vi "Turn Saunders Chamber Off2023.vi"(2 "error in":errorcluster, 3 "Mode":u8 max=2 step=1, 4 "GPIB#":u8=1 max=4 step=1, 5 "GPIB Address":u8=2 max=30 step=1) -> (0 "error out":errorcluster)   [LabVIEW 2023]
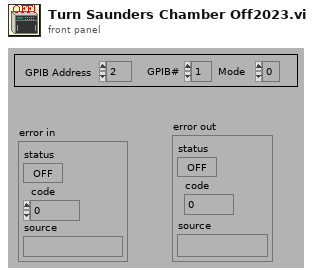
[diagram p1: front panel]
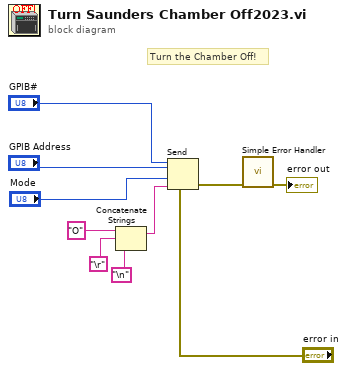
[diagram p0: block diagram]
diagram:
  # "Turn the Chamber Off!"
  n1 = Concatenate Strings("O" ("data string"), "\r", "\n") -> (w3:string)
  n2 = Send(0:"GPIB#", 2:"GPIB Address", 3:"Mode", 4:"error in", 5:w3) -> (8:w7:errorcluster)  [unwired: 2 out]
  n3 = call <vilib>:"Simple Error Handler.vi"("error in (no error)"=w7) -> ("error out"=→"error out":errorcluster)  [unwired: 4 in, 4 out]
